vi "2022 InitGlobalConstants.vi"(8 "error in (no error)":errorcluster, 11 "localConstantSpreadSheet":string[][](array[string])) -> (0 "error out":errorcluster)   [LabVIEW 2020]
uses:
  <vilib>/Rock Robotics/WPI/ThirdParty/Phoenix-LabVIEW/Motor Controller/Controls/CTRE_Phoenix_MotorControl_ControlMode.ctl
  2022 Robot Global Data.vi
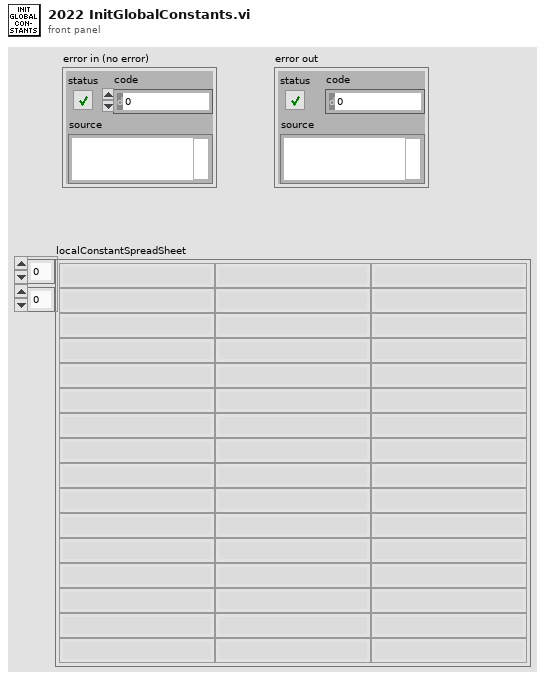
[diagram p1: front panel]
types:
  T1 = cluster{"P Gain":dbl, "I Gain":dbl, "D Gain":dbl, "F Gain":dbl, "I Zone":dbl, "Min Output":dbl, "Max Output":dbl}
  T2 = typedef "CTRE_Phoenix_MotorControl_ControlMode.ctl" = u16
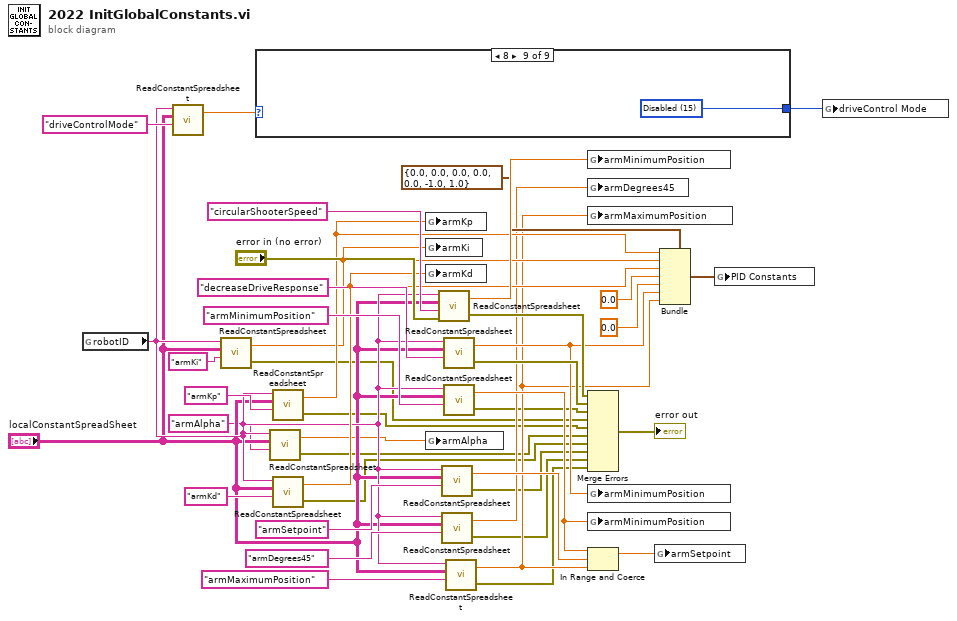
[diagram p0: block diagram]
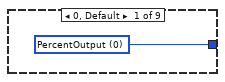
[diagram p2: hidden frame]
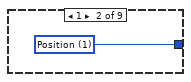
[diagram p3: hidden frame]
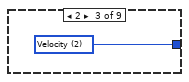
[diagram p4: hidden frame]
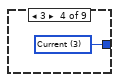
[diagram p5: hidden frame]
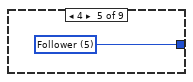
[diagram p6: hidden frame]
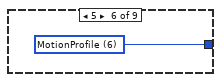
[diagram p7: hidden frame]
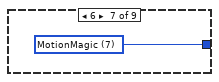
[diagram p8: hidden frame]
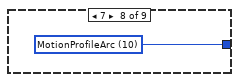
[diagram p9: hidden frame]
diagram:
  n1 = global read "2022 Robot Global Data.vi" "robotID"() -> (w13:string)
  n2 = call "ReadConstantSpreadsheet.vi"("Constant"="driveControlMode", "2022ConstantSpreadSheet"="localConstantSpreadSheet", "Robot ID"=w13) -> ("Constant Value"=w36:dbl)  [unwired: 1 in, 1 out]
  n3 = call "ReadConstantSpreadsheet.vi"("Constant"="armKi", "2022ConstantSpreadSheet"="localConstantSpreadSheet", "Robot ID"=w13) -> ("error out"=w8:errorcluster, "Constant Value"=w22:dbl)  [unwired: 1 in]
  n4 = case shown="8" w36 {
    tunnel: [w43 w44 w45 w46 w47 w48 w49 w50 w51] -> w34
    frame 0, Default {
      w43 = T2 0 items=["PercentOutput"=0, "Position"=1, "Velocity"=2, "Current"=3, "Follower"=5, "MotionProfile"=6, "MotionMagic"=7, "MotionProfileArc"=10, "Disabled"=15] ("driveControl Mode")
    }
    frame 1 {
      w44 = T2 1 items=["PercentOutput"=0, "Position"=1, "Velocity"=2, "Current"=3, "Follower"=5, "MotionProfile"=6, "MotionMagic"=7, "MotionProfileArc"=10, "Disabled"=15] ("driveControl Mode")
    }
    frame 2 {
      w45 = T2 2 items=["PercentOutput"=0, "Position"=1, "Velocity"=2, "Current"=3, "Follower"=5, "MotionProfile"=6, "MotionMagic"=7, "MotionProfileArc"=10, "Disabled"=15] ("driveControl Mode")
    }
    frame 3 {
      w46 = T2 3 items=["PercentOutput"=0, "Position"=1, "Velocity"=2, "Current"=3, "Follower"=5, "MotionProfile"=6, "MotionMagic"=7, "MotionProfileArc"=10, "Disabled"=15] ("driveControl Mode")
    }
    frame 4 {
      w47 = T2 5 items=["PercentOutput"=0, "Position"=1, "Velocity"=2, "Current"=3, "Follower"=5, "MotionProfile"=6, "MotionMagic"=7, "MotionProfileArc"=10, "Disabled"=15] ("driveControl Mode")
    }
    frame 5 {
      w48 = T2 6 items=["PercentOutput"=0, "Position"=1, "Velocity"=2, "Current"=3, "Follower"=5, "MotionProfile"=6, "MotionMagic"=7, "MotionProfileArc"=10, "Disabled"=15] ("driveControl Mode")
    }
    frame 6 {
      w49 = T2 7 items=["PercentOutput"=0, "Position"=1, "Velocity"=2, "Current"=3, "Follower"=5, "MotionProfile"=6, "MotionMagic"=7, "MotionProfileArc"=10, "Disabled"=15] ("driveControl Mode")
    }
    frame 7 {
      w50 = T2 10 items=["PercentOutput"=0, "Position"=1, "Velocity"=2, "Current"=3, "Follower"=5, "MotionProfile"=6, "MotionMagic"=7, "MotionProfileArc"=10, "Disabled"=15] ("driveControl Mode")
    }
    frame 8 {
      w51 = T2 15 items=["PercentOutput"=0, "Position"=1, "Velocity"=2, "Current"=3, "Follower"=5, "MotionProfile"=6, "MotionMagic"=7, "MotionProfileArc"=10, "Disabled"=15] ("driveControl Mode")
    }
  }
  n5 = call "ReadConstantSpreadsheet.vi"("Constant"="armAlpha", "2022ConstantSpreadSheet"="localConstantSpreadSheet", "Robot ID"=w13) -> ("error out"=w5:errorcluster, "Constant Value"=w10:dbl)  [unwired: 1 in]
  n6 = call "ReadConstantSpreadsheet.vi"("Constant"="armKp", "2022ConstantSpreadSheet"="localConstantSpreadSheet", "Robot ID"=w13) -> ("error out"=w7:errorcluster, "Constant Value"=w23:dbl)  [unwired: 1 in]
  n7 = call "ReadConstantSpreadsheet.vi"("Constant"="armKd", "2022ConstantSpreadSheet"="localConstantSpreadSheet", "Robot ID"=w13) -> ("error out"=w4:errorcluster, "Constant Value"=w21:dbl)  [unwired: 1 in]
  n8 = global write "2022 Robot Global Data.vi" "armKp"(w23) -> ()
  n9 = global write "2022 Robot Global Data.vi" "armKi"(w22) -> ()
  n10 = global write "2022 Robot Global Data.vi" "armKd"(w21) -> ()
  n11 = global write "2022 Robot Global Data.vi" "armAlpha"(w10) -> ()
  n12 = call "ReadConstantSpreadsheet.vi"("error in"="error in (no error)", "Constant"="circularShooterSpeed", "2022ConstantSpreadSheet"="localConstantSpreadSheet", "Robot ID"=w13) -> ("error out"=w38:errorcluster, "Constant Value"=w40:dbl)
  n13 = call "ReadConstantSpreadsheet.vi"("Constant"="armSetpoint", "2022ConstantSpreadSheet"="localConstantSpreadSheet", "Robot ID"=w13) -> ("error out"=w3:errorcluster, "Constant Value"=w29:dbl)  [unwired: 1 in]
  n14 = call "ReadConstantSpreadsheet.vi"("Constant"="armDegrees45", "2022ConstantSpreadSheet"="localConstantSpreadSheet", "Robot ID"=w13) -> ("error out"=w2:errorcluster, "Constant Value"=w14:dbl)  [unwired: 1 in]
  n15 = call "ReadConstantSpreadsheet.vi"("Constant"="decreaseDriveResponse", "2022ConstantSpreadSheet"="localConstantSpreadSheet", "Robot ID"=w13) -> ("error out"=w37:errorcluster, "Constant Value"=w19:dbl)  [unwired: 1 in]
  n16 = call "ReadConstantSpreadsheet.vi"("Constant"="armMinimumPosition", "2022ConstantSpreadSheet"="localConstantSpreadSheet", "Robot ID"=w13) -> ("error out"=w9:errorcluster, "Constant Value"=w25:dbl)  [unwired: 1 in]
  n17 = call "ReadConstantSpreadsheet.vi"("Constant"="armMaximumPosition", "2022ConstantSpreadSheet"="localConstantSpreadSheet", "Robot ID"=w13) -> ("error out"=w1:errorcluster, "Constant Value"=w18:dbl)  [unwired: 1 in]
  n18 = global write "2022 Robot Global Data.vi" "armMinimumPosition"(w40) -> ()
  n19 = global write "2022 Robot Global Data.vi" "armDegrees45"(w14) -> ()
  n20 = global write "2022 Robot Global Data.vi" "armMaximumPosition"(w18) -> ()
  n21 = Merge Errors(w38, w37, w9, w8, w7, w5, w4, w3, w2, w1) -> (→"error out":errorcluster)
  n22 = global write "2022 Robot Global Data.vi" "armMinimumPosition"(w19) -> ()
  n23 = global write "2022 Robot Global Data.vi" "armMinimumPosition"(w25) -> ()
  n24 = In Range and Coerce(upper limit=w25, x=w29, lower limit=w18) -> (coerced(x)=w28:dbl)  [unwired: 1 out]
  n25 = global write "2022 Robot Global Data.vi" "armSetpoint"(w28) -> ()
  n26 = Bundle(cluster=T1 {"P Gain"=0.0, "I Gain"=0.0, "D Gain"=0.0, "F Gain"=0.0, "I Zone"=0.0, "Min Output"=-1.0, "Max Output"=1.0} ("PID Constants"), "P Gain"=w23, "I Gain"=w22, "D Gain"=w21, "F Gain"=0.0, "I Zone"=0.0, "Min Output"=w19, "Max Output"=w18) -> (w16:T1)
  n27 = global write "2022 Robot Global Data.vi" "PID Constants"(w16) -> ()
  n28 = global write "2022 Robot Global Data.vi" "driveControl Mode"(w34) -> ()
